vi "4 Axis - Stop.vi"(4 "error in (no error)":errorcluster, 7 "Controller Reference":refnum<k7>) -> (0 "error out":errorcluster, 3 "Controller Reference out":refnum<k7>)   [LabVIEW 2015]
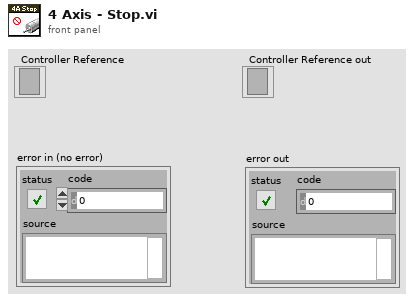
[diagram p1: front panel]
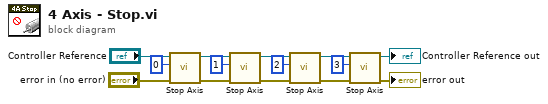
[diagram p0: block diagram]
diagram:
  n1 = call "Stop Axis.vi"("error in (no error)"="error in (no error)", "Axis In"=i16 0, "Controller Reference"="Controller Reference") -> ("error out"=w13:errorcluster, "Controller Reference out"=w14:refnum<k7>)  [unwired: 2 in, 1 out]
  n2 = call "Stop Axis.vi"("error in (no error)"=w13, "Axis In"=i16 1, "Controller Reference"=w14) -> ("error out"=w11:errorcluster, "Controller Reference out"=w12:refnum<k7>)  [unwired: 2 in, 1 out]
  n3 = call "Stop Axis.vi"("error in (no error)"=w11, "Axis In"=i16 2, "Controller Reference"=w12) -> ("error out"=w9:errorcluster, "Controller Reference out"=w10:refnum<k7>)  [unwired: 2 in, 1 out]
  n4 = call "Stop Axis.vi"("error in (no error)"=w9, "Axis In"=i16 3, "Controller Reference"=w10) -> ("error out"=→"error out":errorcluster, "Controller Reference out"=→"Controller Reference out":refnum<k7>)  [unwired: 2 in, 1 out]
